vi "Build Label Properties.vi"(8 "error in (no error)":errorcluster, 10 "Labels":T1 {"scheduleBuildUnit" items=["Millisecond", "Microsecond"]}) -> (0 "error out":errorcluster, 2 "name":string, 4 "Prop Names":string[](array[string]), 6 "Prop Values":variant[](array[variant]))   [LabVIEW 2016, in "Ballard Arinc-429 System Explorer.lvlib"]
uses:
  Ballard Arinc-429 System Explorer.lvlib
  Shared/Controls and Global/Global.vi
  Shared/Ballard Arinc-429 Shared.lvlib
  Controls/Ballard_Label.ctl
  Controls/ARINCParam.ctl
  Controls/Ballard_Word.ctl
  Shared/Controls and Global/TransferType.ctl
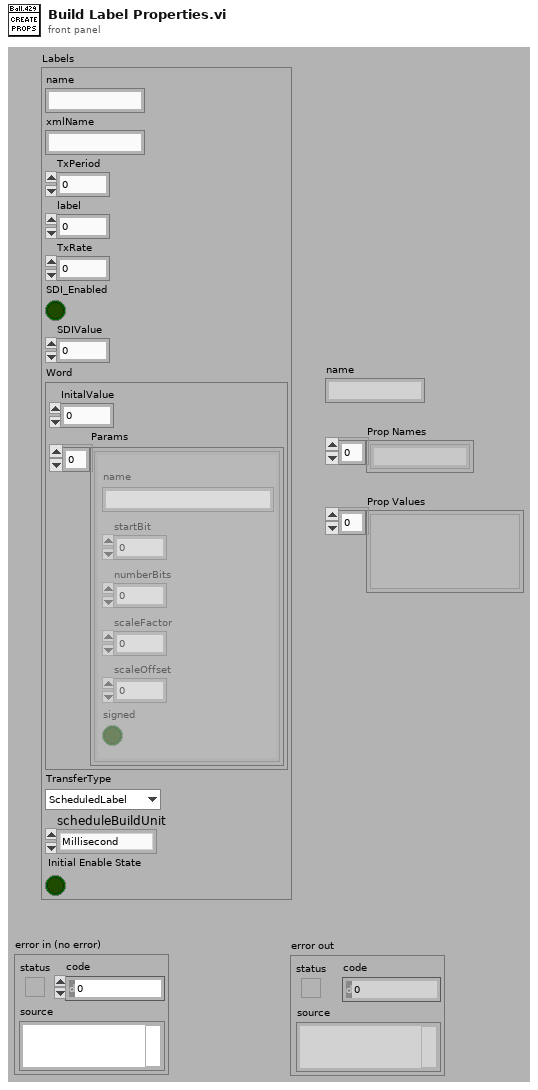
[diagram p1: front panel]
types:
  T1 = typedef "Ballard Arinc-429 System Explorer.lvlib/Ballard_Label.ctl" = cluster{"name":string, "xmlName":string, "TxPeriod":u32, "label":u32, "TxRate":dbl, "SDI_Enabled":bool, "SDIValue":u8, "Word":T2, "TransferType":T4, "scheduleBuildUnit":i32, "Initial Enable State":bool}
  T2 = typedef "Ballard Arinc-429 System Explorer.lvlib/Ballard_Word.ctl" = cluster{"InitalValue":u32, "Params":T3[]}
  T3 = typedef "Ballard Arinc-429 System Explorer.lvlib/ARINCParam.ctl" = cluster{"name":string, "startBit":i32, "numberBits":i32, "scaleFactor":dbl, "scaleOffset":dbl, "signed":bool}
  T4 = typedef "Ballard Arinc-429 Shared.lvlib/TransferType.ctl" = enum16{"ScheduledLabel", "Acyclic", "Block", "Strobe"}
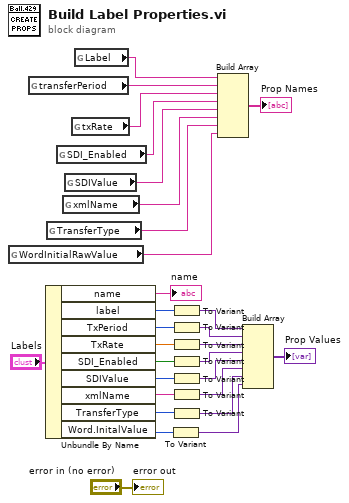
[diagram p0: block diagram]
diagram:
  n1 = global read "Global.vi" "WordInitialRawValue"() -> (w1:string)
  n2 = global read "Global.vi" "transferPeriod"() -> (w21:string)
  n3 = Unbundle By Name("Labels") -> ("name"=→"name":string, "label"=w22:u32, "TxPeriod"=w28:u32, "TxRate"=w18:dbl, "SDI_Enabled"=w13:bool, "SDIValue"=w9:u8, "xmlName"=w6:string, "TransferType"=w4:T4, "Word.InitalValue"=w3:u32)
  n4 = global read "Global.vi" "TransferType"() -> (w8:string)
  n5 = global read "Global.vi" "SDI_Enabled"() -> (w15:string)
  n6 = global read "Global.vi" "xmlName"() -> (w10:string)
  n7 = global read "Global.vi" "SDIValue"() -> (w14:string)
  n8 = global read "Global.vi" "txRate"() -> (w16:string)
  n9 = global read "Global.vi" "Label"() -> (w20:string)
  n10 = To Variant(anything=w3) -> (Variant=w2:variant)
  n11 = To Variant(anything=w22) -> (Variant=w25:variant)
  n12 = To Variant(anything=w28) -> (Variant=w24:variant)
  n13 = To Variant(anything=w18) -> (Variant=w17:variant)
  n14 = To Variant(anything=w13) -> (Variant=w12:variant)
  n15 = To Variant(anything=w9) -> (Variant=w11:variant)
  n16 = To Variant(anything=w6) -> (Variant=w5:variant)
  n17 = To Variant(anything=w4) -> (Variant=w7:variant)
  n18 = Build Array(w20, w21, w16, w15, w14, w10, w8, w1) -> (→"Prop Names":string[])
  n19 = Build Array(w25, w24, w17, w12, w11, w5, w7, w2) -> (→"Prop Values":variant[])
  "error out" <- "error in (no error)"
